vi "Read Export Setting from File.vi"(8 "error in (no error)":errorcluster) -> (0 "error out":errorcluster)   [LabVIEW 2015, in "ConfigHelper.lvlib"]
uses:
  ConfigHelper.lvlib
  Control_Export Setup.ctl
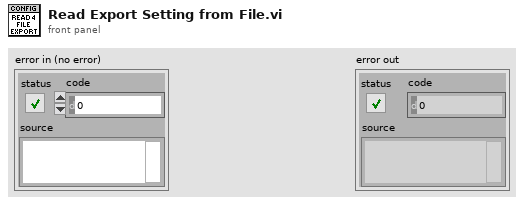
[diagram p1: front panel]
types:
  T1 = typedef "ConfigHelper.lvlib/Control_Export Setup.ctl" = cluster{"Device Name":string, "Export CSV":bool, "Export TDMS":bool, "Export RAW TDMS":bool, "Channel Names":string[]}
  T2 = typedef "PointValueMap.lvlib/PointMap.ctl" = refnum<data-value>
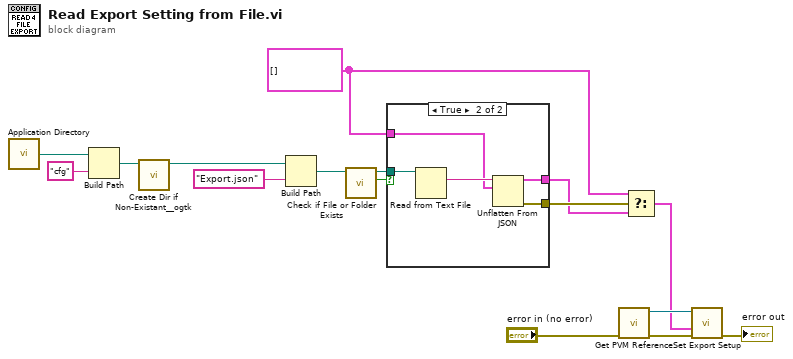
[diagram p0: block diagram]
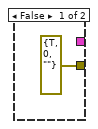
[diagram p2: hidden frame]
diagram:
  w3 = T1[] []
  n1 = call <vilib>:"Application Directory.vi"() -> ("Application Directory"=w16:path)
  n2 = Build Path(base path=w16, name or relative path="cfg") -> (appended path=w14:path)
  n3 = call <userlib>:"Create Dir if Non-Existant__ogtk.vi"("Directory Path"=w14) -> ("dup Directory Path"=w13:path)  [unwired: 8 in, 2 out]
  n4 = Build Path(base path=w13, name or relative path="Export.json") -> (appended path=w11:path)
  n5 = call <vilib>:"Check if File or Folder Exists.vi"("path"=w11) -> ("file or folder exists?"=w10:bool, "dup path"=w9:path)  [unwired: 8 in, 1 out]
  n6 = case shown="True" w10 {
    tunnel: w9 -> [_ w22]
    tunnel: [_ w20] -> w2
    tunnel: [errorcluster {"status"=TRUE, "code"=0, "source"=""} ("error constant") w19] -> w8
    tunnel: w3 -> [_ w18]
    frame False {
    }
    frame True {
      n7 = Read from Text File(file (use dialog)=w22) -> (text=w21:string)  [unwired: 3 in, 3 out]
      n8 = Unflatten From JSON(JSON string=w21, type and defaults=w18) -> (value=w20:T1[], error out=w19:errorcluster)  [unwired: 5 in]
    }
  }
  n9 = call "Get PVM Reference.vi"("error in (no error)"="error in (no error)") -> ("error out"=w6:errorcluster, "Map Out"=w7:T2)  [unwired: 9 in]
  n10 = Select(t=w3, s=w8, f=w2) -> (s? t:f=w1:T1[])
  n11 = call "Set Export Setup.vi"("error in (no error)"=w6, "Export Setup"=w1, "Map"=w7) -> ("error out"=→"error out":errorcluster)  [unwired: 7 in, 1 out]
